vi "UtilityLib.show help.vi"(0 "helpType":T1) -> ()   [LabVIEW 2014, in "UtilityLib.lvlib"]
doc: "Gets the help text on a specific subject like \"help on menus...\"), by looking for text that is surrounded by a specific keyword. The keywords have the following format.\n\nSUBJECTHelpStart\nblabla\nSUBJECTHelpStop\n\nThe keyword SUBJECT may have the following values\nmenu: to be used, to obtain help on the menus and options\ndescription: to be used, to obtain a description of the program\nspecial0: user specific\nspecial1: user specific\nspecial2: user specific\n\nThere exist also two other help types:\nunknown: returns the full description of the calling VI\nabout: returns the full description of the owning library of the calling VI"
uses:
  UtilityLib.lvlib
  UtilityLib.helpType.ctl
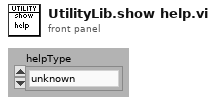
[diagram p1: front panel]
types:
  T1 = typedef "UtilityLib.lvlib/UtilityLib.helpType.ctl" = enum16{"unknown", "menu", "description", "about", "special0", "special1", "special2"}
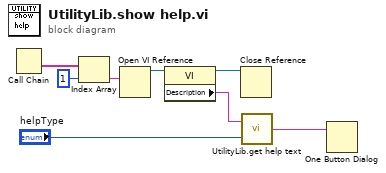
[diagram p0: block diagram]
diagram:
  n1 = Call Chain() -> (call chain=w3:string[])
  n2 = Index Array(array=w3, index=1) -> (element=w5:string)
  n3 = Open VI Reference(vi path=w5) -> (vi reference=w6:refnum<vi>)  [unwired: 5 in, 1 out]
  n4 = property class="VI"(reference=w6) -> (reference out=w7:refnum<vi>, "Description"=w2:string)  [unwired: 1 in, 1 out]
  n5 = Close Reference(reference=w7) -> ()  [unwired: 1 in, 1 out]
  n6 = call "UtilityLib.get help text.vi"("helpType"="helpType", "VIDescription"=w2) -> ("helpText"=w1:string)
  n7 = One Button Dialog(message=w1) -> ()  [unwired: 1 in, 1 out]
